vi "Generate Stream Event.vi"(7 "Direction":T1, 8 "error in (no error)":errorcluster, 10 "Bytes":u8[](array[numeric]) format="%02x", 11 "DebuggingTerminal in":refnum<class "DebuggingTerminal.lvclass">) -> (0 "error out":errorcluster, 3 "DebuggingTerminal out":refnum<class "DebuggingTerminal.lvclass">)   [LabVIEW 2013, in "MQTT Base.lvlib" / "DebuggingTerminal.lvclass"]
uses:
  DebuggingTerminal.lvclass
  Stream Direction -- enum.ctl
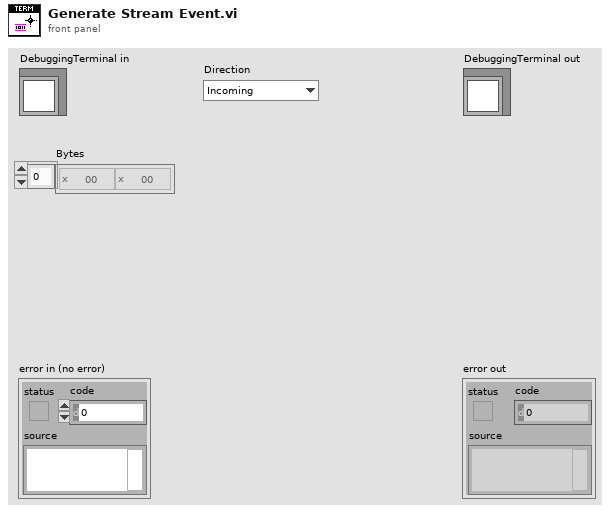
[diagram p1: front panel]
types:
  T1 = typedef "MQTT Base.lvlib/DebuggingTerminal.lvclass/Stream Direction -- enum.ctl" = enum16{"Incoming", "Outgoing"}
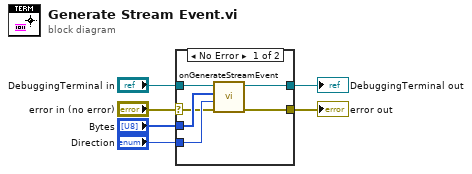
[diagram p0: block diagram]
diagram:
  n1 = case shown="No Error" "error in (no error)" {
    selector: "error in (no error)" -> [w8 w14]
    tunnel: [w7 w14] -> w5
    tunnel: [w9 w13] -> w3
    tunnel: "DebuggingTerminal in" -> [w10 w13]
    tunnel: "Bytes" -> [w12 _]
    tunnel: "Direction" -> [w11 _]
    frame No Error {
      n2 = call-dynamic "onGenerateStreamEvent.vi"("error in (no error)"=w8, "Direction"=w11, "Bytes"=w12, "DebuggingTerminal in"=w10) -> ("error out"=w7:errorcluster, "DebuggingTerminal out"=w9:refnum<class "DebuggingTerminal.lvclass">)  [unwired: 6 in]
    }
    frame Error {
    }
  }
  "error out" <- w5
  "DebuggingTerminal out" <- w3
